vi "LINX - Thermistor Read.vi"() -> ()   [LabVIEW 2020]
doc: "Read one the value of one analog channel from a LINX device."
uses:
  vi.lib/MakerHub/LINX/Private/Type Defs/Temperature Units.ctl
  vi.lib/MakerHub/LINX/Public/Utilities/Open Serial.vi
  vi.lib/MakerHub/LINX/LMH-LINX.lvlib
  vi.lib/MakerHub/LINX/Private/Device/Device.lvlib
panel:
  in  "Temp Units":T1
  in  "Paired Resistance":i32
  in  "AI Channel":u8
  in  "Analog Ref Voltage":dbl
  out "Loop Rate (Hz)":u32
  in  "Stop Button":bool
  out "Analog Data":dbl(graph)
  in  "Serial Port":refnum<visa-resource-name>
  # "Circuit Schematic"
  # "LINX Device Settings"
  # "Temperature"
  # "LINX - Thermistor Read Example\n\nThis example demonstrates how to read from a thermistor attached to an analog input\n\nInstructions\n1. Select the COM Port associated with the LINX Device.\n2. Select the Analog Channel to read.\n3. Click the Run Arrow."
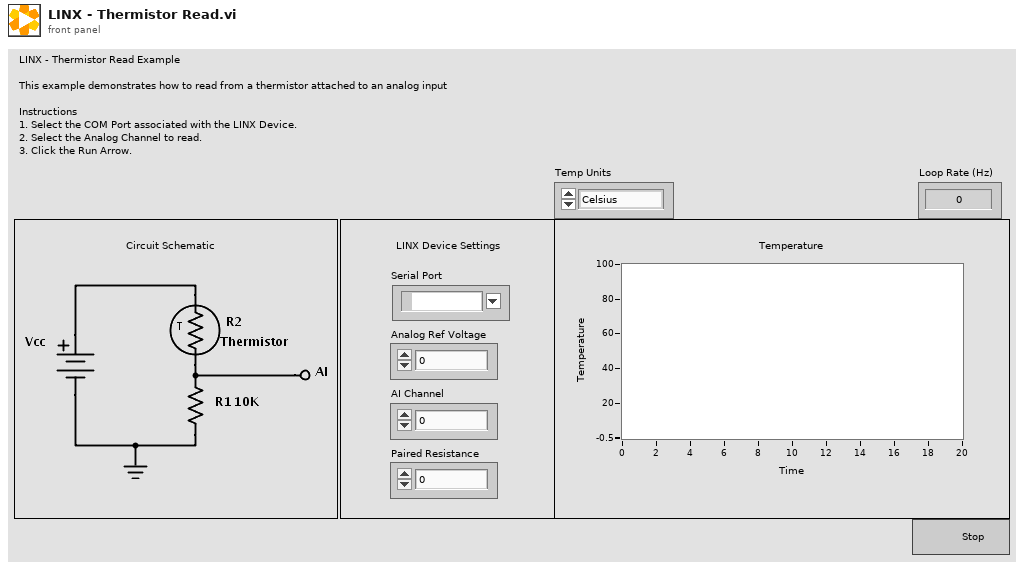
[diagram p1: front panel]
types:
  T1 = typedef "LMH-LINX.lvlib/Temperature Units.ctl" = enum16{"Celsius", "Fahrenheit", "Kelvin", "Rankine"}
  T2 = typedef "LMH-LINX.lvlib/LINX Ref.ctl" = cluster{"IO":T3, "Interface":T4, "LINX Device Config":T5}
  T3 = typedef "LMH-LINX.lvlib/Platform.ctl" = enum16{"Remote", "Local"}
  T4 = typedef "LMH-LINX.lvlib/Interface.ctl" = enum16{"Serial", "TCP"}
  T5 = typedef "Device.lvlib/LINX Device Config.ctl" = cluster{"Interface":T4, "COM Port":refnum<visa-resource-name>, "TCP Configuration":T6, "Device Family":u8, "Device ID":u8, "Device Name":string, "TCP Ref":refnum<k5>, "Channels":T7}
  T6 = typedef "Device.lvlib/TCP Config.ctl" = cluster{"IP Address":string, "Port":u16}
  T7 = typedef "LMH-LINX.lvlib/Channels.ctl" = cluster{"DI":u8[], "DO":u8[], "AI":u8[], "AO":u8[], "PWM":u8[], "QE":u8[], "UART":u8[], "I2C 2":u8[], "SPI":u8[], "CAN":u8[], "Servo":u8[], "AI Ref (V)":dbl, "AI Resolution (Bits)":u8, "AO Ref (V)":dbl, "AO Resolution (Bits)":u8}
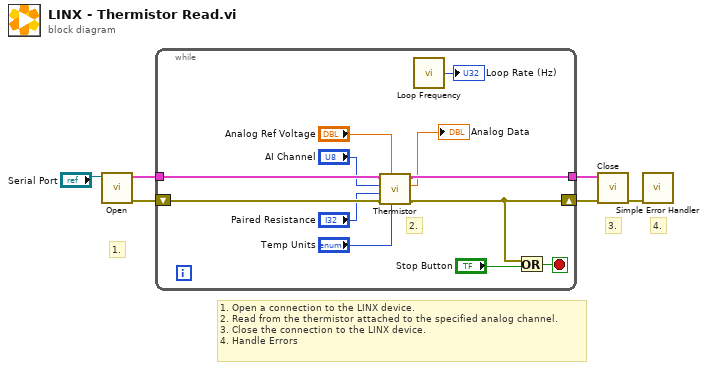
[diagram p0: block diagram]
diagram:
  # "1. Open a connection to the LINX device.\n2. Read from the thermistor attached to the specified analog channel.\n3. Close the connection to the LINX device.\n4. Handle Errors"
  # "4."
  # "3."
  # "1."
  n1 = call-poly "Open.vi"("Serial Port"="Serial Port") -> ("Error Out"=w5:errorcluster, "LINX Resource"=w6:T2)  [unwired: 8 in, 1 out]
  n2 = while {
    tunnel: w6 -> [w15]
    tunnel: [w14] -> w4
    shift-right: [w13] -> w3
    shift-left: w5 -> [w12]
    stop <- w18 stop-if-true
    # "2."
    n3 = call "Thermistor.vi"("Units (C)"="Temp Units", "Analog Ref Override"="Analog Ref Voltage", "Error In"=w12, "Paired Resistance"="Paired Resistance", "AI Channel"="AI Channel", "LINX Resource"=w15) -> ("Error Out"=w13:errorcluster, "Temperature"=→"Analog Data":dbl, "LINX Resource"=w14:T2)  [unwired: 3 in]
    n4 = call "Loop Frequency.vi"() -> ("Loop Rate (Hz)"=→"Loop Rate (Hz)":u32)
    n5 = Or(x=w13, y="Stop Button") -> (x .or. y?=w18:bool)
  }
  n6 = call "Close.vi"("Error In"=w3, "LINX Resource"=w4) -> ("Error Out"=w1:errorcluster)  [unwired: 9 in]
  n7 = call <vilib>:"Simple Error Handler.vi"("error in (no error)"=w1) -> ()  [unwired: 4 in, 5 out]
